vi "LVIS_ReadConfig.vi"(8 "Error In":errorcluster) -> (0 "Error Out":errorcluster, 3 "Disable":bool)   [LabVIEW 2015]
doc: "Reads in the LVIS_Settings file configuration values and loads them to the appropiate variables."
uses:
  Globals/LVIS_IsGlobal.vi
  <vilib>/Utility/config.llb/Read Key (String).vi
  Globals/LVIS_DcGlobals.vi
  <vilib>/Utility/config.llb/Read Key (Boolean).vi
  <vilib>/Utility/config.llb/NI_LVConfig.lvlib
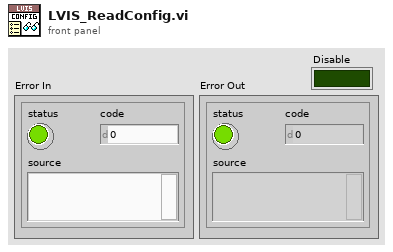
[diagram p1: front panel]
types:
  T1 = typedef "NI_LVConfig.lvlib/Config Data RefNum.ctl" = refnum<k1>
  T2 = cluster{"[0]":string, "[1]":string, "[2]":string, "[3]":string}
  T3 = cluster{"[0]":string, "[1]":string, "[2]":string, "[3]":string, "[4]":string, "[5]":string}
  T4 = cluster{"[0]":string, "[1]":string, "[2]":string, "[3]":string, "[4]":string}
  T5 = cluster{"EventName":string, "EventStart":string, "EventStop":string, "EventStatus":string, "EventClientID":string, "IS_EventID":string, "EventMeta":string, "ProductLine":string, "ProcessName":string, "Station":string, "Operator":string, "SN":string, "Model":string, "Manufacturer":string}
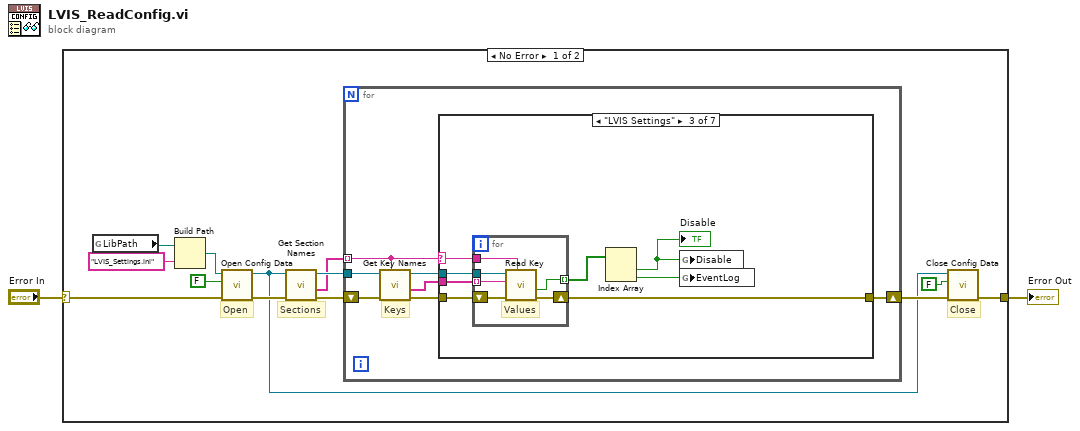
[diagram p0: block diagram]
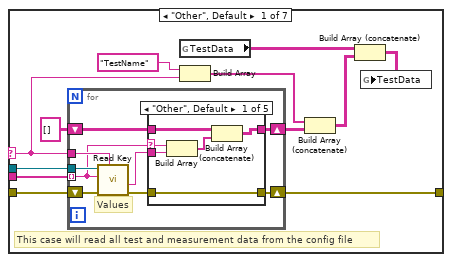
[diagram p2: hidden frame]
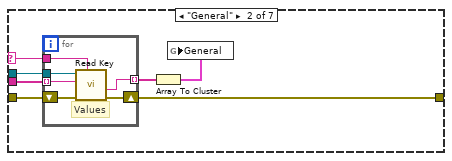
[diagram p7: hidden frame]
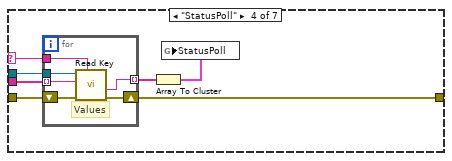
[diagram p8: hidden frame]
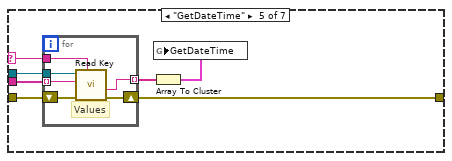
[diagram p9: hidden frame]
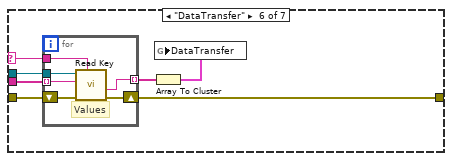
[diagram p10: hidden frame]
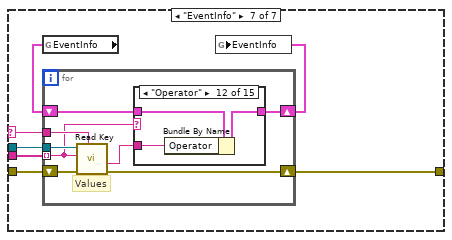
[diagram p11: hidden frame]
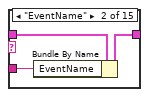
[diagram p13: hidden frame]
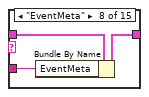
[diagram p19: hidden frame]
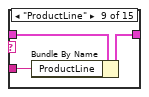
[diagram p20: hidden frame]
diagram:
  n1 = case shown="No Error" "Error In" {
    selector: "Error In" -> [w5 w172]
    tunnel: [w10 w172] -> w1
    frame No Error {
      # "Open"
      # "Close"
      # "Sections"
      n2 = global read "LVIS_IsGlobal.vi" "LibPath"() -> (w7:path)
      n3 = Build Path(base path=w7, name or relative path="LVIS_Settings.ini") -> (appended path=w6:path)
      n4 = call <vilib>:"Open Config Data.vi"("error in (no error)"=w5, "create file if necessary (T)"=FALSE, "configuration file path"=w6) -> ("error out"=w4:errorcluster, "refnum"=w3:T1)  [unwired: 6 in, 1 out]
      n5 = call <vilib>:"Get Section Names.vi"("error in (no error)"=w4, "refnum"=w3) -> ("error out"=w15:errorcluster, "section names"=w13:string[], "refnum out"=w14:T1)  [unwired: 7 in]
      n6 = for {
        shift-right: [w17] -> w12
        shift-left: w15 -> [w22]
        tunnel: w14 -> [w20]
        tunnel: w13 -> [w16] mode=indexing
        # "Keys"
        n7 = call <vilib>:"Get Key Names.vi"("section"=w16, "error in (no error)"=w22, "refnum"=w20) -> ("error out"=w21:errorcluster, "key names"=w18:string[], "refnum out"=w19:T1)  [unwired: 5 in, 1 out]
        n8 = case shown="\"LVIS Settings\"" w16 {
          selector: w16 -> [w30 w61 w75 w88 w101 w114 w127]
          tunnel: w21 -> [w34 w64 w78 w91 w104 w117 w130]
          tunnel: w19 -> [w32 w63 w77 w90 w103 w116 w129]
          tunnel: w18 -> [w33 w62 w76 w89 w102 w115 w128]
          tunnel: [w26 w59 w74 w86 w99 w112 w126] -> w17
          frame "Other", Default {
            # "This case will read all test and measurement data from the config file"
            n9 = for {
              tunnel: w33 -> [w37] mode=indexing
              tunnel: w32 -> [w42]
              tunnel: w30 -> [w41]
              shift-right: [w35] -> w26
              shift-left: w34 -> [w43]
              shift-right: [w38] -> w28
              shift-left: string[][] [] ("appended array") -> [w39]
              # "Values"
              n10 = call-poly <vilib>:"Read Key.vi"("section"=w41, "error in (no error)"=w43, "key"=w37, "refnum"=w42) -> ("error out"=w36:errorcluster, "value"=w40:string)  [unwired: 4 in, 2 out]
              n11 = case shown="\"Other\", Default" w37 {
                selector: w37 -> [w45 _ _ _ _]
                tunnel: w40 -> [w49 _ _ _ _]
                tunnel: w39 -> [w48 w51 w53 w55 w57]
                tunnel: [w46 w51 w53 w55 w57] -> w38
                tunnel: w36 -> [w44 w50 w52 w54 w56]
                tunnel: [w44 w50 w52 w54 w56] -> w35
                frame "Other", Default {
                  n12 = Build Array(w45, w49) -> (w47:string[])
                  n13 = Build Array (concatenate)(w48, w47) -> (w46:string[][])
                }
                frame "TestDateTime" {
                  # "Ignore TestDT"
                }
                frame "TestStatus" {
                  # "Ignore TestStatus"
                }
                frame "TestClientID" {
                  # "Ignore TestClientID"
                }
                frame "IS_TestID" {
                  # "Ignore IS_TestID"
                }
              }
            }
            n14 = global read "LVIS_IsGlobal.vi" "TestData"() -> (w27:string[][][])
            n15 = Build Array("TestName" ("element"), w30) -> (w29:string[])
            n16 = Build Array (concatenate)(w29, w28) -> (w25:string[][])
            n17 = Build Array (concatenate)(w27, w25) -> (w24:string[][][])
            n18 = global write "LVIS_IsGlobal.vi" "TestData"(w24) -> ()
          }
          frame "General" {
            n19 = for {
              shift-right: [w66] -> w59
              shift-left: w64 -> [w70]
              tunnel: w63 -> [w69]
              tunnel: w62 -> [w68] mode=indexing
              tunnel: w61 -> [w67]
              tunnel: [w65] -> w60 mode=indexing
              # "Values"
              n20 = call-poly <vilib>:"Read Key.vi"("section"=w67, "error in (no error)"=w70, "key"=w68, "refnum"=w69) -> ("error out"=w66:errorcluster, "value"=w65:string)  [unwired: 4 in, 2 out]
            }
            n21 = Array To Cluster(array=w60) -> (cluster=w58:T2)
            n22 = global write "LVIS_DcGlobals.vi" "General"(w58) -> ()
          }
          frame "LVIS Settings" {
            n23 = for {
              shift-right: [w80] -> w74
              shift-left: w78 -> [w84]
              tunnel: w77 -> [w83]
              tunnel: w76 -> [w82] mode=indexing
              tunnel: w75 -> [w81]
              tunnel: [w79] -> w73 mode=indexing
              # "Values"
              n24 = call-poly <vilib>:"Read Key.vi"("section"=w81, "error in (no error)"=w84, "key"=w82, "refnum"=w83) -> ("error out"=w80:errorcluster, "value"=w79:bool)  [unwired: 4 in, 2 out]
            }
            n25 = Index Array(array=w73) -> (element #1=w71:bool, element #2=w72:bool)  [unwired: 2 in]
            "Disable" <- w71
            n26 = global write "LVIS_DcGlobals.vi" "Disable"(w71) -> ()
            n27 = global write "LVIS_DcGlobals.vi" "EventLog"(w72) -> ()
          }
          frame "StatusPoll" {
            n28 = for {
              shift-right: [w93] -> w86
              shift-left: w91 -> [w97]
              tunnel: w90 -> [w96]
              tunnel: w89 -> [w95] mode=indexing
              tunnel: w88 -> [w94]
              tunnel: [w92] -> w87 mode=indexing
              # "Values"
              n29 = call-poly <vilib>:"Read Key.vi"("section"=w94, "error in (no error)"=w97, "key"=w95, "refnum"=w96) -> ("error out"=w93:errorcluster, "value"=w92:string)  [unwired: 4 in, 2 out]
            }
            n30 = Array To Cluster(array=w87) -> (cluster=w85:T3)
            n31 = global write "LVIS_DcGlobals.vi" "StatusPoll"(w85) -> ()
          }
          frame "GetDateTime" {
            n32 = for {
              shift-right: [w106] -> w99
              shift-left: w104 -> [w110]
              tunnel: w103 -> [w109]
              tunnel: w102 -> [w108] mode=indexing
              tunnel: w101 -> [w107]
              tunnel: [w105] -> w100 mode=indexing
              # "Values"
              n33 = call-poly <vilib>:"Read Key.vi"("section"=w107, "error in (no error)"=w110, "key"=w108, "refnum"=w109) -> ("error out"=w106:errorcluster, "value"=w105:string)  [unwired: 4 in, 2 out]
            }
            n34 = Array To Cluster(array=w100) -> (cluster=w98:T4)
            n35 = global write "LVIS_DcGlobals.vi" "GetDateTime"(w98) -> ()
          }
          frame "DataTransfer" {
            n36 = for {
              shift-right: [w119] -> w112
              shift-left: w117 -> [w123]
              tunnel: w116 -> [w122]
              tunnel: w115 -> [w121] mode=indexing
              tunnel: w114 -> [w120]
              tunnel: [w118] -> w113 mode=indexing
              # "Values"
              n37 = call-poly <vilib>:"Read Key.vi"("section"=w120, "error in (no error)"=w123, "key"=w121, "refnum"=w122) -> ("error out"=w119:errorcluster, "value"=w118:string)  [unwired: 4 in, 2 out]
            }
            n38 = Array To Cluster(array=w113) -> (cluster=w111:T4)
            n39 = global write "LVIS_DcGlobals.vi" "DataTransfer"(w111) -> ()
          }
          frame "EventInfo" {
            n40 = global read "LVIS_IsGlobal.vi" "EventInfo"() -> (w125:T5)
            n41 = for {
              shift-right: [w135] -> w126
              shift-left: w130 -> [w138]
              tunnel: w129 -> [w137]
              tunnel: w128 -> [w131] mode=indexing
              tunnel: w127 -> [w136]
              shift-right: [w133] -> w124
              shift-left: w125 -> [w134]
              # "Values"
              n42 = call-poly <vilib>:"Read Key.vi"("section"=w136, "error in (no error)"=w138, "key"=w131, "refnum"=w137) -> ("error out"=w135:errorcluster, "value"=w132:string)  [unwired: 4 in, 2 out]
              n43 = case shown="\"Operator\"" w131 {
                tunnel: w134 -> [w139 w142 w143 w144 w145 w146 w147 w150 w153 w156 w159 w162 w165 w168 w171]
                tunnel: [w139 w141 w143 w144 w145 w146 w147 w149 w152 w155 w158 w161 w164 w167 w170] -> w133
                tunnel: w132 -> [_ w140 _ _ _ _ _ w148 w151 w154 w157 w160 w163 w166 w169]
                frame "Unknown", Default {
                }
                frame "EventName" {
                  n44 = Bundle By Name(cluster=w142, "EventName"=w140) -> (w141:T5)
                }
                frame "EventStart" {
                  # "Ignore EventStart"
                }
                frame "EventStop" {
                  # "Ignore EventStop"
                }
                frame "EventStatus" {
                  # "Ignore EventStatus"
                }
                frame "EventClientID" {
                  # "Ignore EventClientID"
                }
                frame "IS_EventID" {
                  # "Ignore IS_EventID"
                }
                frame "EventMeta" {
                  n45 = Bundle By Name(cluster=w150, "EventMeta"=w148) -> (w149:T5)
                }
                frame "ProductLine" {
                  n46 = Bundle By Name(cluster=w153, "ProductLine"=w151) -> (w152:T5)
                }
                frame "ProcessName" {
                  n47 = Bundle By Name(cluster=w156, "ProcessName"=w154) -> (w155:T5)
                }
                frame "Station" {
                  n48 = global write "LVIS_IsGlobal.vi" "Station"(w157) -> ()
                  n49 = Bundle By Name(cluster=w159, "Station"=w157) -> (w158:T5)
                }
                frame "Operator" {
                  n50 = Bundle By Name(cluster=w162, "Operator"=w160) -> (w161:T5)
                }
                frame "SN" {
                  n51 = Bundle By Name(cluster=w165, "SN"=w163) -> (w164:T5)
                }
                frame "Model" {
                  n52 = Bundle By Name(cluster=w168, "Model"=w166) -> (w167:T5)
                }
                frame "Manufacturer" {
                  n53 = Bundle By Name(cluster=w171, "Manufacturer"=w169) -> (w170:T5)
                }
              }
            }
            n54 = global write "LVIS_IsGlobal.vi" "EventInfo"(w124) -> ()
          }
        }
      }
      n55 = call <vilib>:"Close Config Data.vi"("error in (no error)"=w12, "write file if changed (T)"=FALSE, "refnum"=w3) -> ("error out"=w10:errorcluster)  [unwired: 7 in, 1 out]
    }
    frame Error {
    }
  }
  "Error Out" <- w1
